vi "Create Enhanced Config JSON.vi"(11 "Value":variant) -> (0 "error out":errorcluster, 3 "PAtools JSON":string)   [LabVIEW 2023]
uses:
  Plugin/AMS Power Supply Template/Configuration Params.ctl
  <vilib>/ADAS Replay HIL/Template Node/Plugin/Template Node/Common Configuration Params.ctl
  Capabilities/Capabilities/High Level Capabilities/Power Supply Cluster/Power Supply Cluster.lvclass
  Capabilities/Capabilities/Utilities/Utilities.lvlib
  <vilib>/ADAS Replay HIL/AdasCommonUtilities/AdasCommonUtilities.lvlib
  <vilib>/ADAS Replay HIL/Template Node/Plugin/Template Node/Template Node.lvclass
  Plugin/AMS Power Supply Template/AMS Power Supply Template.lvclass
panel:
  in  "Default Parameters":T1={"Common"={"Iteration Interval (s)"=0.001, "T0 (ns)"=0, "Priority"=100, "Processor"=-2, "Wait in Ready State"=TRUE}, "Amount of Channels"=0, "Address"="localhost"} {"Common"."Iteration Interval (s)" format="%#_13g"}
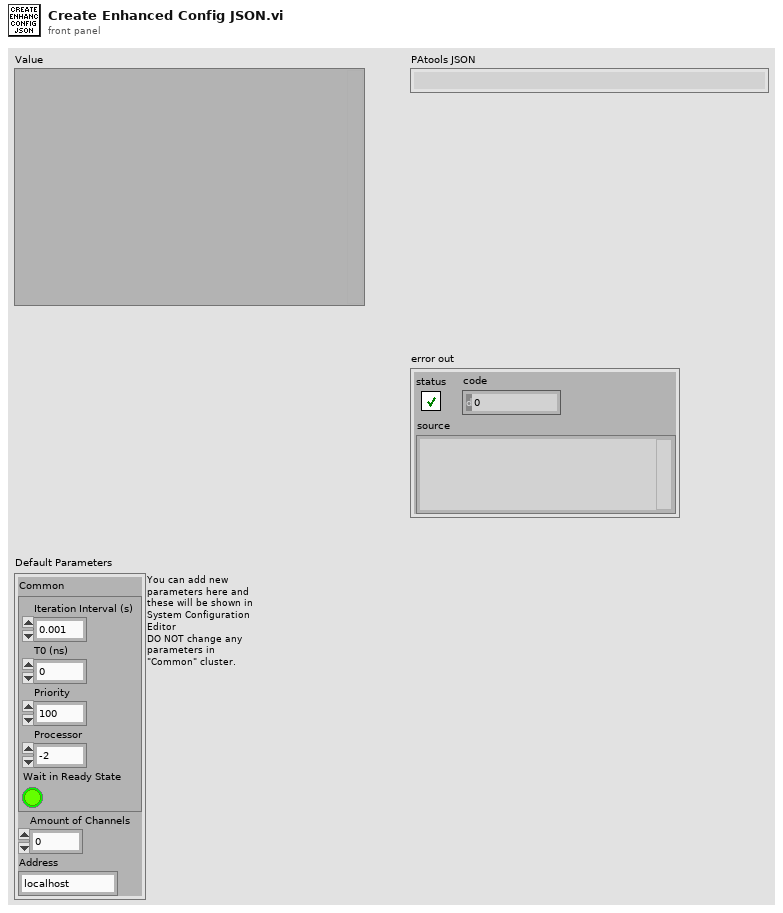
[diagram p1: front panel]
types:
  T1 = typedef "AMS Power Supply Template.lvlib/AMS Power Supply Template.lvclass/Configuration Params.ctl" = cluster{"Common":T2, "Amount of Channels":u32, "Address":string}
  T2 = typedef "Template Node.lvlib/Template Node.lvclass/Common Configuration Params.ctl" = cluster{"Iteration Interval (s)":dbl, "T0 (ns)":u64, "Priority":i32, "Processor":i32, "Wait in Ready State":bool}
  T3 = typedef "NI_App_Builder_API.lvlib/Build Specification Version.ctl" = cluster{"Major":u16, "Minor":u16, "Fix":u16, "Build":u16}
  T4 = typedef "Utilities.lvlib/Channel.ctl" = cluster{"Title":string, "SubTitle":string[], "Consumer?":bool, "Name":string, "Description":string, "Size":i32, "OffSets":i32[], "DataType":string[], "DefaultValue":dbl[]}
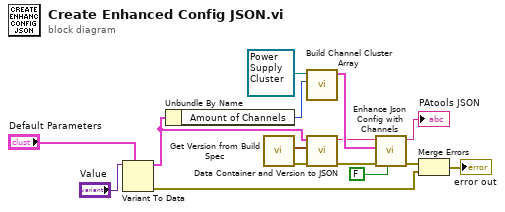
[diagram p0: block diagram]
diagram:
  n1 = Variant To Data(type="Default Parameters", Variant="Value") -> (data=w7:T1, error out=w4:errorcluster)  [unwired: 1 in]
  n2 = Unbundle By Name(w7) -> ("Amount of Channels"=w14:u32)
  n3 = call "Get Version from Build Spec.vi"() -> ("error out"=w5:errorcluster, "Version"=w13:T3)  [unwired: 8 in, 2 out]
  n4 = call-dynamic "Build Channel Cluster Array.vi"("Power Supply Cluster.lvclass in"=refnum<class "Power Supply Cluster.lvclass"> refnum ("Power Supply Cluster.lvclass"), "Channels Amount"=w14) -> ("Channels out"=w15:cluster{"Channels":T4[]})  [unwired: 8 in]
  n5 = call <vilib>:"Data Container and Version to JSON.vi"("error in (no error)"=w5, "Version"=w13, "Container Variant"=w7) -> ("error out"=w10:errorcluster, "JSON string"=w12:string)  [unwired: 7 in]
  n6 = call "Enhance Json Config with Channels.vi"("Save PAtools config Json? (Default: True)"=FALSE ("Save PAtools config Json?"), "error in"=w10, "Channels"=w15, "Json Config"=w12) -> ("error out"=w3:errorcluster, "PAtools JSON"=→"PAtools JSON":string)  [unwired: 6 in]
  n7 = Merge Errors(w3, w4) -> (→"error out":errorcluster)
